vi "PhotonUtils_GetDistanceToPose.vi"(10 "TargetPose":T1={"TRANSLATION"={"X"=0.0, "Y"=0.0}, "ROTATION"={"VALUE"=0.0, "COS"=1.0, "SIN"=0.0}} {"ROTATION"."SIN" format="%13.4f"; "ROTATION"."COS" format="%13.4f"; "ROTATION"."VALUE" format="%13.4f"; "TRANSLATION"."Y" format="%14.3f"; "TRANSLATION"."X" format="%14.3f"}, 11 "RobotPose":T1={"TRANSLATION"={"X"=0.0, "Y"=0.0}, "ROTATION"={"VALUE"=0.0, "COS"=1.0, "SIN"=0.0}} {"ROTATION"."SIN" format="%13.4f"; "ROTATION"."COS" format="%13.4f"; "ROTATION"."VALUE" format="%13.4f"; "TRANSLATION"."Y" format="%14.3f"; "TRANSLATION"."X" format="%14.3f"}) -> (3 "DistanceToPose":dbl)   [LabVIEW 2019, in "PhotonVisionLib.lvlib"]
doc: "Returns the distance between two poses\n\nInputs:\n - RobotPose -- Pose2d of the robot.\n - TargetPose -- Pose2d of the target\n\nOutputs\n - DistanceToPose -- The calculated distance between the poses."
uses:
  PhotonVisionLib.lvlib
  <vilib>/Rock Robotics/WPI/ThirdParty/JAS_Junk/TrajLib/Trajectory_Library.lvlib
  <vilib>/Rock Robotics/WPI/ThirdParty/JAS_Junk/TrajLib/TypeDef/TRANSLATION2D.ctl
  <vilib>/Rock Robotics/WPI/ThirdParty/JAS_Junk/TrajLib/TypeDef/ROTATION2D.ctl
  <vilib>/Rock Robotics/WPI/ThirdParty/JAS_Junk/TrajLib/TypeDef/POSE2D.ctl
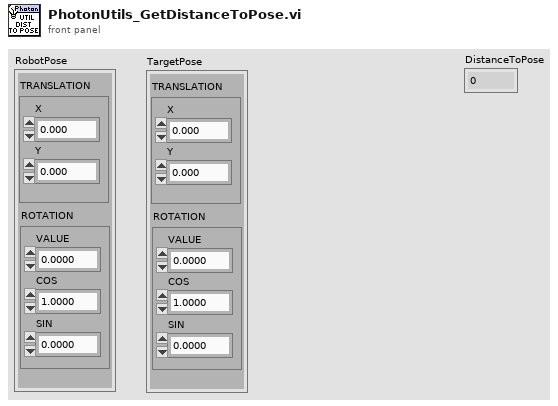
[diagram p1: front panel]
types:
  T1 = typedef "Trajectory_Library.lvlib/POSE2D.ctl" = cluster{"TRANSLATION":T2, "ROTATION":T3}
  T2 = typedef "Trajectory_Library.lvlib/TRANSLATION2D.ctl" = cluster{"X":dbl, "Y":dbl}
  T3 = typedef "Trajectory_Library.lvlib/ROTATION2D.ctl" = cluster{"VALUE":dbl, "COS":dbl, "SIN":dbl}
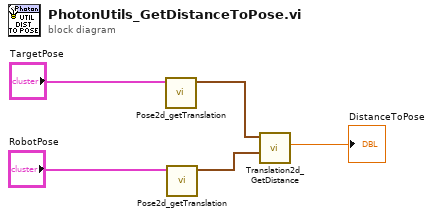
[diagram p0: block diagram]
diagram:
  n1 = call <vilib>:"Pose2d_getTranslation.vi"("in POSE"="TargetPose") -> ("outTRANSLATION"=w3:T2)  [unwired: 10 in]
  n2 = call <vilib>:"Pose2d_getTranslation.vi"("in POSE"="RobotPose") -> ("outTRANSLATION"=w2:T2)  [unwired: 10 in]
  n3 = call <vilib>:"Translation2d_GetDistance.vi"("other Translation"=w2, "In Translation"=w3) -> ("Distance"=→"DistanceToPose":dbl)  [unwired: 9 in]
